vi "Create Section View Data U16.vi"(8 "error in":errorcluster, 10 "Image U16":u16[][](array[numeric]), 11 "Graph with Section Views in":refnum<class "Graph with Section Views.lvclass">) -> (0 "error out":errorcluster, 1 "Cursor Column Data":cluster{"Image U16":u16[], "Array":u16[]}, 2 "Cursor Row Data":cluster{"Array":u16[], "Image U16":u16[]})   [LabVIEW 2025, in "Graph with Section Views.lvclass"]
uses:
  Graph with Section Views.lvclass
  Base Graph/Base Graph.lvclass/Base Graph.ctl
  <vilib>/Analysis/1siggen.llb/Ramp Pattern by Delta.vi
  Base Graph/Base Graph.lvclass
  <vilib>/Analysis/NI_AALBase.lvlib
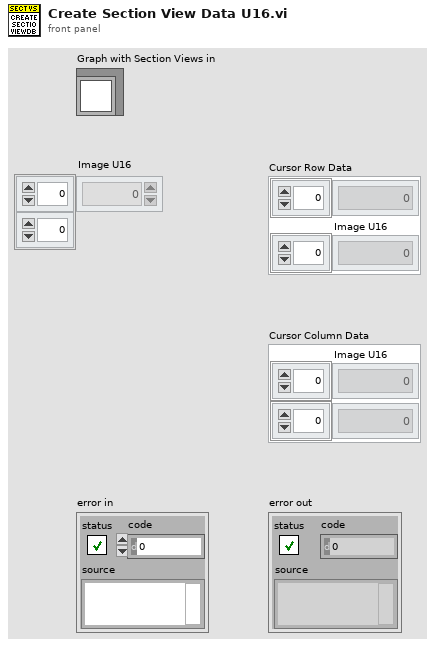
[diagram p1: front panel]
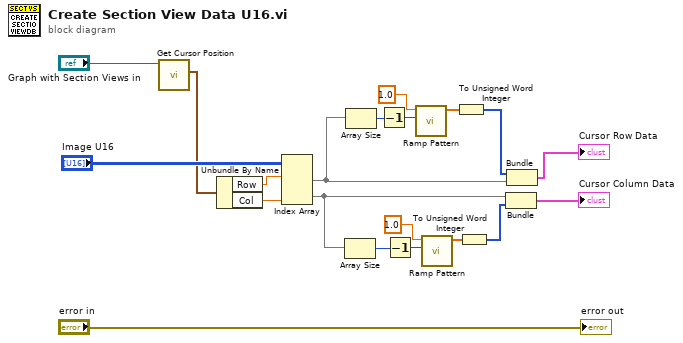
[diagram p0: block diagram]
diagram:
  n1 = call "Get Cursor Position.vi"("Base Graph in"="Graph with Section Views in") -> ("Cursor Position"=w17:cluster{"Col":dbl, "Row":dbl})  [unwired: 9 in, 1 out]
  n2 = Unbundle By Name(w17) -> ("Row"=w16:dbl, "Col"=w15:dbl)
  n3 = Index Array(array="Image U16", index (row) #1=w16, index (col) #2=w15) -> (element #1=w11:u16[], element #2=w1:u16[])  [unwired: 2 in]
  n4 = Array Size(array=w1) -> (size(s)=w9:i32)
  n5 = Array Size(array=w11) -> (size(s)=w13:i32)
  n6 = Decrement(x=w13) -> (x-1=w12:i32)
  n7 = Decrement(x=w9) -> (x-1=w8:i32)
  n8 = call-poly <vilib>:"Ramp Pattern.vi"("end"=w12, "delta"=1.0) -> ("Ramp Pattern"=w5:dbl[])  [unwired: 7 in, 2 out]
  n9 = call-poly <vilib>:"Ramp Pattern.vi"("end"=w8, "delta"=1.0) -> ("Ramp Pattern"=w7:dbl[])  [unwired: 7 in, 2 out]
  n10 = To Unsigned Word Integer(number=w5) -> (unsigned 16bit integer=w4:u16[])
  n11 = To Unsigned Word Integer(number=w7) -> (unsigned 16bit integer=w6:u16[])
  n12 = Bundle("Image U16"=w1, w6) -> (→"Cursor Column Data":cluster{"Image U16":u16[], u16[]})  [unwired: 1 in]
  n13 = Bundle(w4, "Image U16"=w11) -> (→"Cursor Row Data":cluster{u16[], "Image U16":u16[]})  [unwired: 1 in]
  "error out" <- "error in"
